vi "TEST - Get All Control Values {Variant}.vi"(8 "error in (no error)":errorcluster) -> (0 "error out":errorcluster, 2 "pass":bool)   [LabVIEW 2009]
uses:
  <userlib>/_OpenG.lib/lvdata/lvdata.llb/Type Descriptor Enumeration__ogtk.ctl
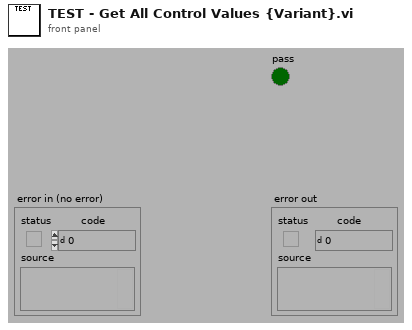
[diagram p1: front panel]
types:
  T1 = typedef "Type Descriptor Enumeration__ogtk.ctl" = enum8{"<Null>", "I8", "I16", "I32", "I64", "U8", "U16", "U32", "U64", "SGL", "DBL", "EXT", "CSG", "CDB", "CXT", "0x0F", "0x10", "0x11", "0x12", "0x13", "0x14", "Enum U8", "Enum U16", "Enum U32", "Enum U64", "SGL PQ", "DBL PQ", "EXT PQ", "CSG PQ", "CDB PQ", "CXT PQ", "0x1F", "0x20", "Boolean", "0x22", "0x23", "0x24", "0x25", "0x26", "0x27", "0x28", "0x29", "0x2A", "0x2B", "0x2C", "0x2D", "0x2E", "0x2F", "String", "0x31", "Path", "Pict", "0x34", "0x35", "0x36", "DAQ", "0x38", "0x39", "0x3A", "0x3B", "0x3C", "0x3D", "0x3E", "0x3F", "Array", "0x41", "0x42", "0x43", "0x44", "0x45", "0x46", "0x47", "0x48", "0x49", "0x4A", "0x4B", "0x4C", "0x4D", "0x4E", "0x4F", "Cluster", "0x51", "0x52", "Variant", "Waveform", "0x55", "0x56", "0x57", "0x58", "0x59", "0x5A", "0x5B", "0x5C", "0x5D", "0x5E", "0x5F", "0x60", "0x61", "0x62", "0x63", "0x64", "0x65", "0x66", "0x67", "0x68", "0x69", "0x6A", "0x6B", "0x6C", "0x6D", "0x6E", "0x6F", "Refnum"}
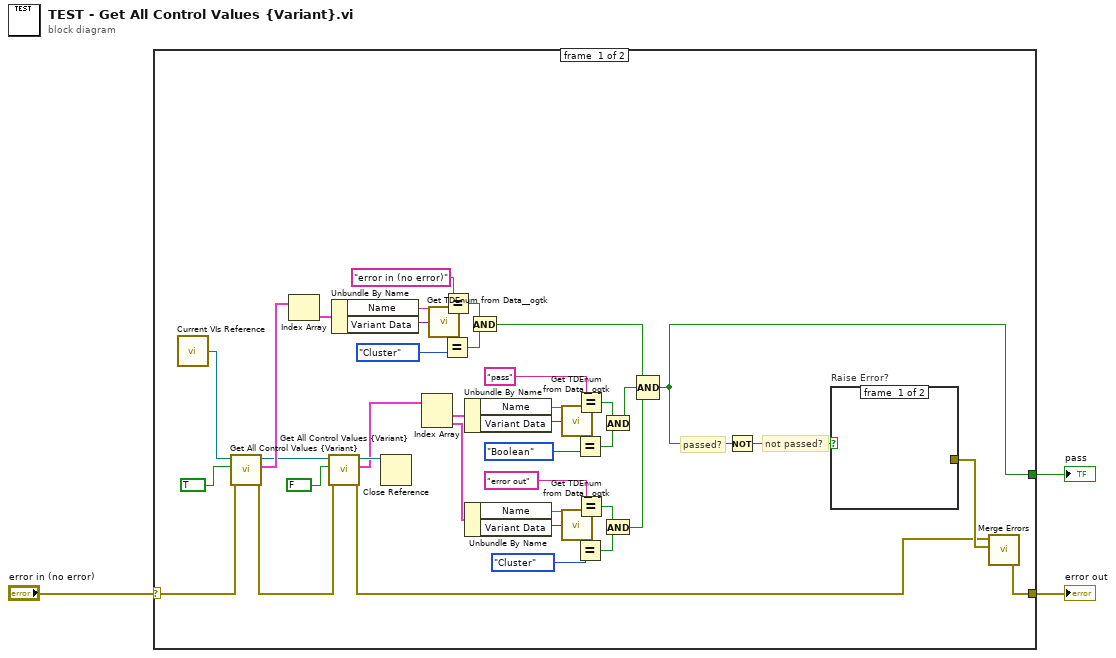
[diagram p0: block diagram]
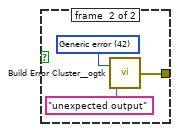
[diagram p2: hidden frame]
diagram:
  n1 = case shown="No Error" "error in (no error)" {
    selector: "error in (no error)" -> [w41 w48]
    tunnel: [w4 _] -> w3
    tunnel: [w44 w48] -> w1
    frame #0 {
      # "not passed?"
      # "passed?"
      n2 = call "Current VIs Reference.vi"() -> ("Current VI's reference"=w39:refnum<vi>)  [unwired: 5 in]
      n3 = call "Get All Control Values {Variant}.vi"("error in (no error)"=w41, "controls (FALSE: indicators)"=TRUE ("controls"), "VI Refnum"=w39) -> ("error out"=w27:errorcluster, "All Control Values"=w38:cluster{"Name":string, "Variant Data":variant}[], "VI Refnum dup"=w29:refnum<vi>)  [unwired: 6 in]
      n4 = Index Array(array=w38) -> (element=w37:cluster{"Name":string, "Variant Data":variant})  [unwired: 1 in]
      n5 = call "Get All Control Values {Variant}.vi"("error in (no error)"=w27, "controls (FALSE: indicators)"=FALSE ("controls"), "VI Refnum"=w29) -> ("error out"=w26:errorcluster, "All Control Values"=w16:cluster{"Name":string, "Variant Data":variant}[], "VI Refnum dup"=w25:refnum<vi>)  [unwired: 6 in]
      n6 = Unbundle By Name(w37) -> ("Name"=w33:string, "Variant Data"=w36:variant)
      n7 = Close Reference(reference=w25) -> ()  [unwired: 1 in, 1 out]
      n8 = Index Array(array=w16) -> (element #1=w17:cluster{"Name":string, "Variant Data":variant}, element #2=w8:cluster{"Name":string, "Variant Data":variant})  [unwired: 2 in]
      n9 = call <userlib>:"Get TDEnum from Data__ogtk.vi"("Data"=w36) -> ("Type Descriptor Enumeration"=w34:T1)  [unwired: 4 in]
      n10 = Equal?(x=w34, y=Type_Descriptor_Enumeration__ogtk."Cluster" ("Type Descriptor Enumeration")) -> (x = y?=w30:bool)
      n11 = Equal?(x="error in (no error)" ("Name"), y=w33) -> (x = y?=w31:bool)
      n12 = Unbundle By Name(w17) -> ("Name"=w21:string, "Variant Data"=w18:variant)
      n13 = Unbundle By Name(w8) -> ("Name"=w12:string, "Variant Data"=w15:variant)
      n14 = And(x=w31, y=w30) -> (x .and. y?=w5:bool)
      n15 = call <userlib>:"Get TDEnum from Data__ogtk.vi"("Data"=w18) -> ("Type Descriptor Enumeration"=w20:T1)  [unwired: 4 in]
      n16 = call <userlib>:"Get TDEnum from Data__ogtk.vi"("Data"=w15) -> ("Type Descriptor Enumeration"=w13:T1)  [unwired: 4 in]
      n17 = Equal?(x=w20, y=Type_Descriptor_Enumeration__ogtk."Boolean" ("Type Descriptor Enumeration")) -> (x = y?=w24:bool)
      n18 = Equal?(x=w13, y=Type_Descriptor_Enumeration__ogtk."Cluster" ("Type Descriptor Enumeration")) -> (x = y?=w9:bool)
      n19 = Equal?(x="pass" ("Name"), y=w21) -> (x = y?=w23:bool)
      n20 = Equal?(x="error out" ("Name"), y=w12) -> (x = y?=w10:bool)
      n21 = And(x=w23, y=w24) -> (x .and. y?=w6:bool)
      n22 = And(x=w10, y=w9) -> (x .and. y?=w7:bool)
      n23 = Compound Arithmetic op=AND(w5, w6, w7) -> (w4:bool)
      n24 = Not(x=w4) -> (.not. x?=w42:bool)
      n25 = case "Raise Error?" shown="True" w42 {
        tunnel: [_ w45] -> w43
        frame #0 {
        }
        frame #1 {
          w46 = 42 items=["No error", "Argument error", "Memory is full", "Out of zone", "End of file", "File already open", "Generic file I/O error", "File not found", "File permission error", "Disk is full", "Duplicate path", "Too many files open", "System feature not enabled", "Resource file not found", "Cannot add resource", "Resource not found", "Image not found", "Image memory error", "Pen does not exist", "Config type invalid", "Config token not found", "Config parse error", "Config memory error", "Bad external code format", "Bad external code offset", "External code not present", "Null window", "Destroy window error", "Null menu", "Print aborted", "Bad print record", "Print driver error", "Windows error during printing", "Memory error during printing", "Print dialog error", "Generic print error", "Invalid device refnum", "Device not found", "Device parameter error", "Device unit error", "Cannot open device", "Device call aborted", "Generic error", "Cancelled by user", "Object ID too low", "Object ID too high", "Object not in heap", "Unknown heap", "Unknown object (invalid DefProc)", "Unknown object (DefProc not in table)", "Message out of range", "Invalid (null) method", "Unknown message", "Manager call not supported", "Bad address", "Network operation in progress", "Network operation timed out", "Connection is busy", "Network attribute not supported", "Network error", "Address in use", "System out of memory", "Connection aborted", "Connection refused", "Not connected", "Already connected", "Connection closed", "Initialization error (interapplication manager)", "Bad occurrence", "Wait on unbound occurrence handler", "Occurrence queue overflow", "Datalog type conflict", "Unused", "Unrecognized type (interapplication manager)", "Memory corrupt", "Failed to make temporary DLL", "Old CIN version", "Drag socket not found", "Failed to load drop-object", "Failed to register OLE object", "Failed to release OLE object", "Format specifier type mismatch", "Unknown format specifier", "Too few format specifiers", "Too many format specifiers", "Scan failed", "Newer CIN version", "Error converting to variant", "Runtime menu error", "Password tampered", "Variant attribute not found", "Incompatible variant data type", "Event data is not available", "Event Store is not present", "Occurrence is not found", "Event Queue is not created", "Event info is not available", "Refnum passed is NULL", "Error retrieving Class GUID", "Error retrieving CoClass GUID", "Error retrieving TypeLib GUID.", "Bad built application magic bytes.", "Specific driver is different from the specific driver associated with the Logical Name.", "There is no session opened to the class driver.", "Max Error", "MAX - Error with config objects", "MAX - Error loading configuration", "MAX - Group not supported"]
          n26 = call <userlib>:"Build Error Cluster__ogtk.vi"("String to Prepend to source (\"\")"="unexpected output" ("String to Prepend to source (\"\")"), "code"=w46) -> ("error out"=w45:errorcluster)
        }
      }
      n27 = call <vilib>:"Merge Errors.vi"("error in 2 (no error)"=w43, "error in 1 (no error)"=w26) -> ("error out"=w44:errorcluster)  [unwired: 5 in]
    }
    frame #1 {
    }
  }
  "pass" <- w3
  "error out" <- w1
